vi "c_Linkboard.vi"() -> (1 "Case Label":T1)   [LabVIEW 2022 SP3, in "ArduinoOperator.lvclass"]
uses:
  <vilib>/addons/_Workers/Library/Case Label.ctl
  ArduinoOperator.lvclass
  ArduinoOperator.lvclass/ArduinoOperator.ctl
  <vilib>/addons/_Workers/Library/Workers.lvlib
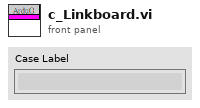
[diagram p1: front panel]
types:
  T1 = typedef "Workers.lvlib/Case Label.ctl" = string
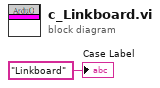
[diagram p0: block diagram]
diagram:
  "Case Label" <- T1 "Linkboard" ("Case Label")
